vi "Terminate.vi"(8 "error in (no error)":errorcluster, 10 "Message in":refnum<class "TerminateMessage.lvclass">=refnum, 11 "Cobolt in":refnum<class "Cobolt.lvclass">=refnum) -> (0 "error out":errorcluster, 3 "Cobolt out":refnum<class "Cobolt.lvclass">)   [LabVIEW 2012, in "Cobolt.lvclass"]
doc: "This member function is called when the statemachine in the run.vi receives an 'terminate' command. It closes the RabbitMQ connection. \n\nOverride this member function in your derived class to release all previously acquired resources (but don't forget to call the parent method). If your component has subcomponents, they count as resources, and you have to release them by calling their own terminate functions."
uses:
  Cobolt.lvclass
  Murmex/LabVIEW/Murmex/TerminateMessage/TerminateMessage.lvclass
panel:
  # "This method is called when the TERMINATE\ntrigger is sent. \n\nOverride this method when your component needs to\nrespond to this trigger. \n\nCall parent for proper implementation"
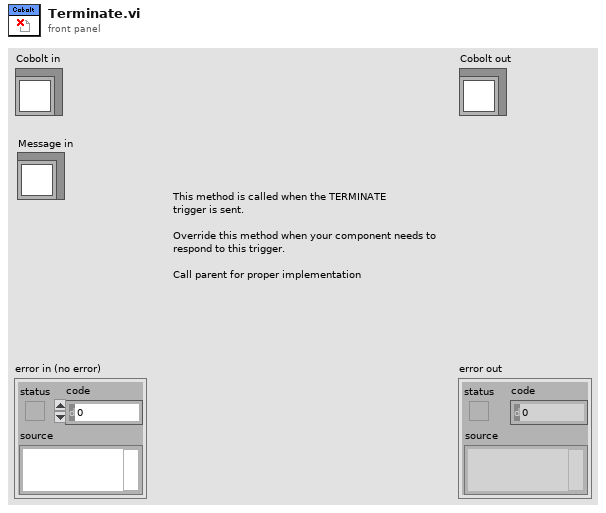
[diagram p1: front panel]
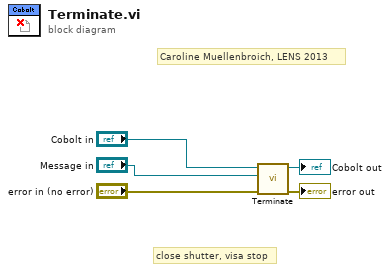
[diagram p0: block diagram]
diagram:
  # "close shutter, visa stop"
  # "Caroline Muellenbroich, LENS 2013"
  n1 = call-parent "Terminate.vi"("error in (no error)"="error in (no error)", "Message in"="Message in", "Murmex in"="Cobolt in") -> ("error out"=→"error out":errorcluster, "Murmex out"=→"Cobolt out":refnum<class "Cobolt.lvclass">)  [unwired: 7 in]
